vi "ConverFileToDiscData.vi"(11 "FileData":u8[](array[numeric])) -> (2 "FileStartIndexOnDisc":i32[](array[numeric]), 3 "DiscData":i64[](array[numeric]))   [LabVIEW 2023, in "2024_9.lvclass"]
uses:
  2024_9.lvclass
  2024_9.lvclass/2024_9.ctl
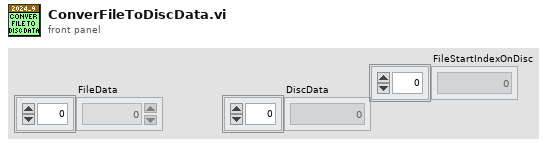
[diagram p1: front panel]
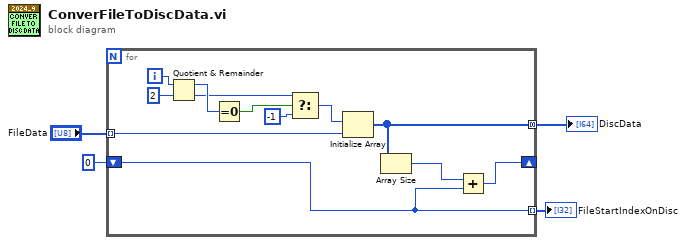
[diagram p0: block diagram]
diagram:
  n1 = for {
    tunnel: [w8] -> w3 mode=concatenating
    tunnel: "FileData" -> [w9] mode=indexing
    shift-right: [w5] -> _
    shift-left: 0 ("y") -> [w7]
    tunnel: [w7] -> w1 mode=indexing
    i -> [w16]
    n2 = Quotient & Remainder(x=w16, y=2) -> (x-y*floor(x/y)=w14:i32, floor(x/y)=w12:i32)
    n3 = Equal To 0?(x=w14) -> (x = 0?=w13:bool)
    n4 = Select(t=w12, s=w13, f=i64 -1) -> (s? t:f=w10:i64)
    n5 = Initialize Array(w10, w9) -> (w8:i64[])
    n6 = Array Size(array=w8) -> (size(s)=w6:i32)
    n7 = Add(x=w6, y=w7) -> (x+y=w5:i32)
  }
  "DiscData" <- w3
  "FileStartIndexOnDisc" <- w1
